vi "red_buoy_threshing_particle.vi"(4 "lum":cluster{"Lower value":i32, "Upper value":i32}={"Lower value"=0, "Upper value"=255}, 5 "hue":cluster{"Lower value":i32, "Upper value":i32}={"Lower value"=7, "Upper value"=14}, 6 "sat":cluster{"Lower value":i32, "Upper value":i32}={"Lower value"=0, "Upper value"=255}, 8 "Image":T1, 9 "error in (no error)":errorcluster) -> (0 "error out":errorcluster, 1 "circular particles":dbl[][](array[numeric]), 3 "Image Out":T1(plugin-control))   [LabVIEW 2009]
uses:
  <vilib>/vision/Image Controls.llb/IMAQ Image.ctl
  <vilib>/vision/NI_Vision_Development_Module.lvlib
panel:
  in  "max circularity":dbl
  out "size(s)":i32[](array[numeric])
  out "Particle Measurements (Pixels)":dbl[][](array[numeric]) format="%.2f"
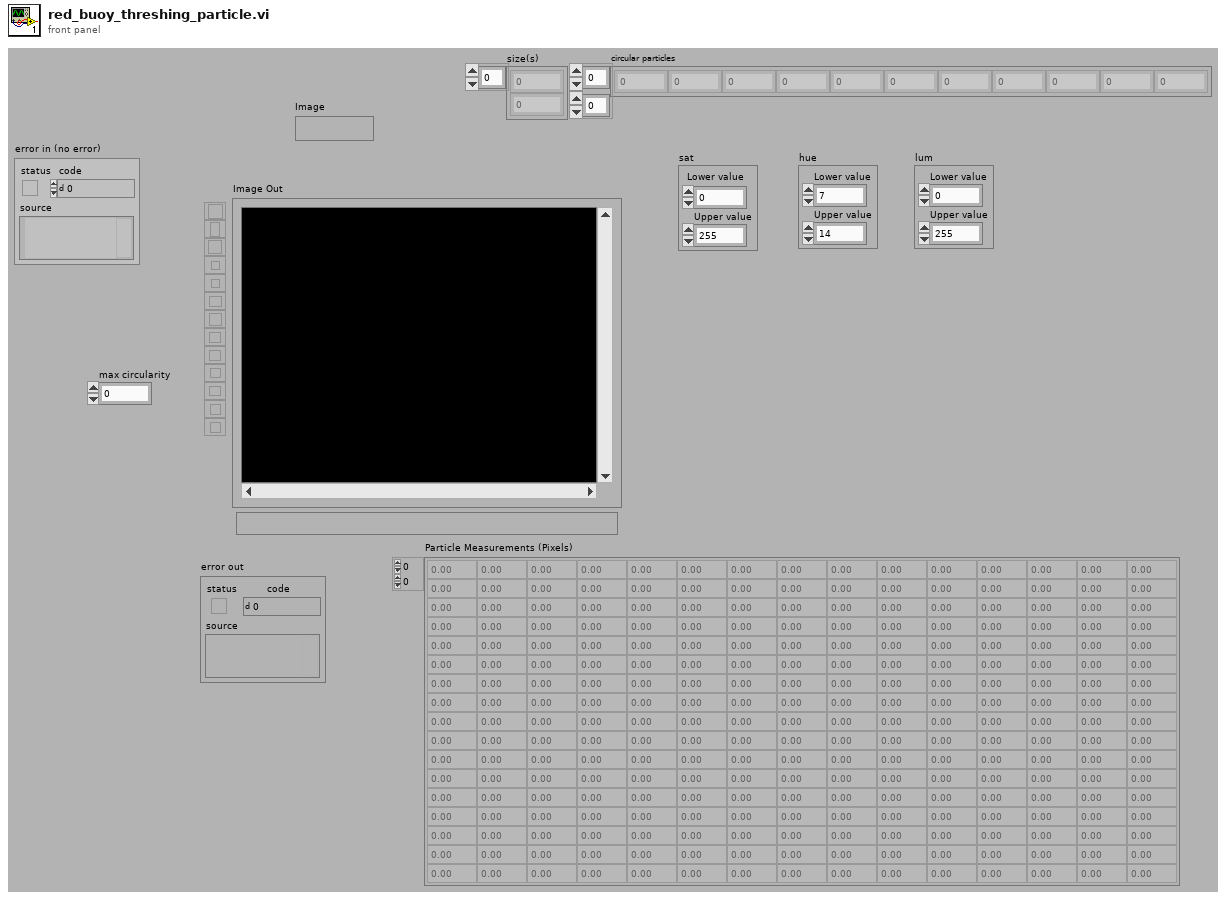
[diagram p1: front panel]
types:
  T1 = typedef "IMAQ Image.ctl" = refnum<image>
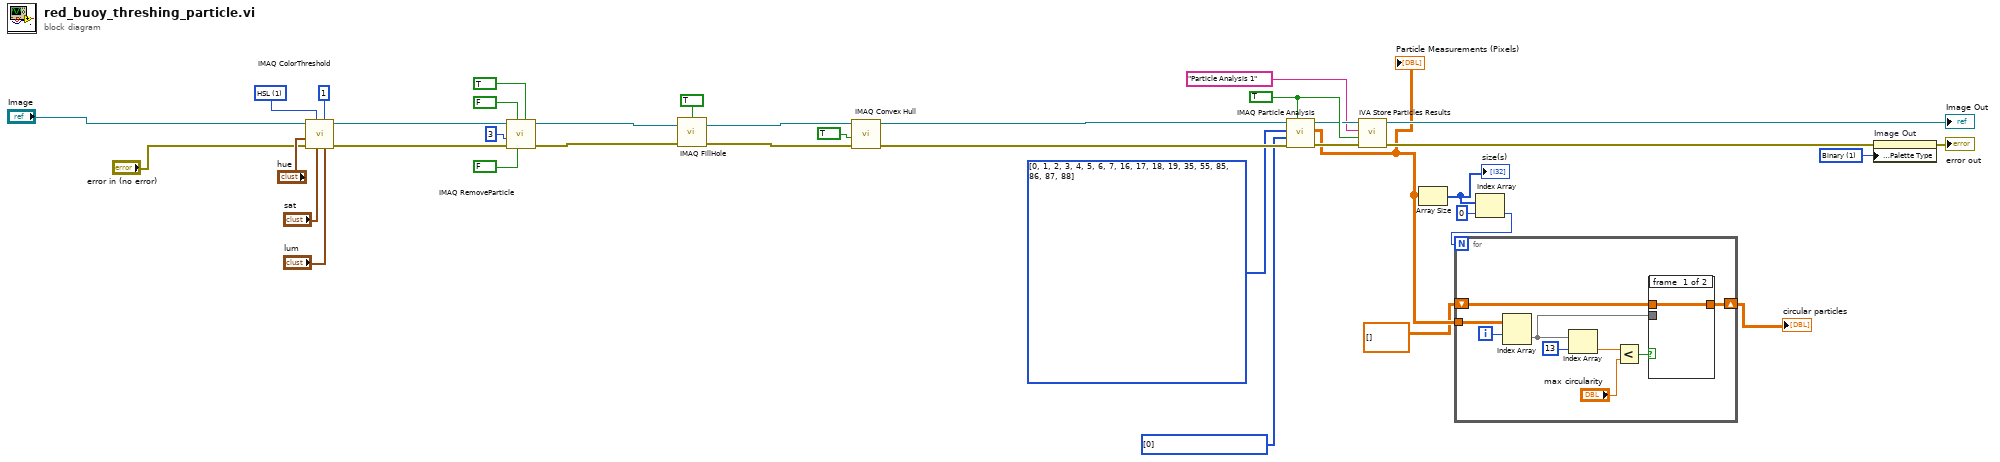
[diagram p0: block diagram]
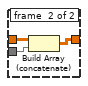
[diagram p2: hidden frame]
diagram:
  w11 = u32 1 items=["Grayscale", "Binary", "Gradient", "Rainbow", "Temperature", "User Defined"] ("Palette")
  w19 = i32[] [0] items=["Center of Mass X", "Center of Mass Y", "First Pixel X", "First Pixel Y", "Bounding Rect Left", "Bounding Rect Top", "Bounding Rect Right", "Bounding Rect Bottom", "Max Feret Diameter Start X", "Max Feret Diameter Start Y", "Max Feret Diameter End X", "Max Feret Diameter End Y", "Max Horiz. Segment Length Left", "Max Horiz. Segment Length Right", "Max Horiz. Segment Length Row", "-", "Bounding Rect Width", "Bounding Rect Height", "Bounding Rect Diagonal", "Perimeter", "Convex Hull Perimeter", "Holes' Perimeter", "Max Feret Diameter", "Equivalent Ellipse Major Axis", "Equivalent Ellipse Minor Axis", "Equivalent Ellipse Minor Axis (Feret)", "Equivalent Rect Long Side", "Equivalent Rect Short Side", "Equivalent Rect Diagonal", "Equivalent Rect Short Side (Feret)", "Average Horiz. Segment Length", "Average Vert. Segment Length", "Hydraulic Radius", "Waddel Disk Diameter", "-", "Area", "Holes' Area", "Particle & Holes' Area", "Convex Hull Area", "Image Area", "-", "Number of Holes", "Number of Horiz. Segments", "Number of Vert. Segments", "-", "Orientation", "Max Feret Diameter Orientation", "-", "% Area/Image Area", "% Area/(Particle & Holes' Area)", "Ratio of Equivalent Ellipse Axes", "Ratio of Equivalent Rect Sides", "-", "Elongation Factor", "Compactness Factor", "Heywood Circularity Factor", "Type Factor", "-", "Sum X", "Sum Y", "Sum XX", "Sum XY", "Sum YY", "Sum XXX", "Sum XXY", "Sum XYY", "Sum YYY", "-", "Moment of Inertia XX", "Moment of Inertia XY", "Moment of Inertia YY", "Moment of Inertia XXX", "Moment of Inertia XXY", "Moment of Inertia XYY", "Moment of Inertia YYY", "Norm. Moment of Inertia XX", "Norm. Moment of Inertia XY", "Norm. Moment of Inertia YY", "Norm. Moment of Inertia XXX", "Norm. Moment of Inertia XXY", "Norm. Moment of Inertia XYY", "Norm. Moment of Inertia YYY", "Hu Moment 1", "Hu Moment 2", "Hu Moment 3", "Hu Moment 4", "Hu Moment 5", "Hu Moment 6", "Hu Moment 7"] ("Real-World Measurements")
  w7 = i32[] [0, 1, 2, 3, 4, 5, 6, 7, 16, 17, 18, 19, 35, 55, 85, 86, 87, 88] items=["Center of Mass X", "Center of Mass Y", "First Pixel X", "First Pixel Y", "Bounding Rect Left", "Bounding Rect Top", "Bounding Rect Right", "Bounding Rect Bottom", "Max Feret Diameter Start X", "Max Feret Diameter Start Y", "Max Feret Diameter End X", "Max Feret Diameter End Y", "Max Horiz. Segment Length Left", "Max Horiz. Segment Length Right", "Max Horiz. Segment Length Row", "-", "Bounding Rect Width", "Bounding Rect Height", "Bounding Rect Diagonal", "Perimeter", "Convex Hull Perimeter", "Holes' Perimeter", "Max Feret Diameter", "Equivalent Ellipse Major Axis", "Equivalent Ellipse Minor Axis", "Equivalent Ellipse Minor Axis (Feret)", "Equivalent Rect Long Side", "Equivalent Rect Short Side", "Equivalent Rect Diagonal", "Equivalent Rect Short Side (Feret)", "Average Horiz. Segment Length", "Average Vert. Segment Length", "Hydraulic Radius", "Waddel Disk Diameter", "-", "Area", "Holes' Area", "Particle & Holes' Area", "Convex Hull Area", "Image Area", "-", "Number of Holes", "Number of Horiz. Segments", "Number of Vert. Segments", "-", "Orientation", "Max Feret Diameter Orientation", "-", "% Area/Image Area", "% Area/(Particle & Holes' Area)", "Ratio of Equivalent Ellipse Axes", "Ratio of Equivalent Rect Sides", "-", "Elongation Factor", "Compactness Factor", "Heywood Circularity Factor", "Type Factor", "-", "Sum X", "Sum Y", "Sum XX", "Sum XY", "Sum YY", "Sum XXX", "Sum XXY", "Sum XYY", "Sum YYY", "-", "Moment of Inertia XX", "Moment of Inertia XY", "Moment of Inertia YY", "Moment of Inertia XXX", "Moment of Inertia XXY", "Moment of Inertia XYY", "Moment of Inertia YYY", "Norm. Moment of Inertia XX", "Norm. Moment of Inertia XY", "Norm. Moment of Inertia YY", "Norm. Moment of Inertia XXX", "Norm. Moment of Inertia XXY", "Norm. Moment of Inertia XYY", "Norm. Moment of Inertia YYY", "Hu Moment 1", "Hu Moment 2", "Hu Moment 3", "Hu Moment 4", "Hu Moment 5", "Hu Moment 6", "Hu Moment 7"] ("Pixel Measurements")
  w17 = TRUE ("Connectivity 4/8 (8)")
  w36 = u16 1 items=["RGB", "HSL", "HSV", "HSI"] ("Color Mode")
  n1 = call "IMAQ ColorThreshold"("Blue or Luma or Val or Inten Range"="lum", "Replace Value"=1, "Green or Sat Range"="sat", "Color Mode"=w36, "error in (no error)"="error in (no error)", "Red or Hue Range"="hue", "Image Src"="Image") -> ("error out"=w32:errorcluster, "Image Dst Out"=w27:T1)  [unwired: 1 in, 2 out]
  n2 = call "IMAQ RemoveParticle"("Connectivity 4/8 (8)"=TRUE, "Low Pass/High Pass (Low)"=FALSE, "Square/Hexa (Square)"=FALSE, "error in (no error)"=w32, "Number of Erosion"=3, "Image Src"=w27) -> ("error out"=w26:errorcluster, "Image Dst Out"=w24:T1)  [unwired: 1 in, 3 out]
  n3 = call "IMAQ FillHole"("error in (no error)"=w26, "Image Src"=w24, "Connectivity 4/8 (8)"=TRUE) -> ("error out"=w23:errorcluster, "Image Dst Out"=w22:T1)  [unwired: 1 in, 2 out]
  n4 = call "IMAQ Convex Hull"("error in (no error)"=w23, "Connectivity 4/8 (8)"=TRUE, "Image Src"=w22) -> ("error out"=w20:errorcluster, "Image Dst Out"=w18:T1)  [unwired: 1 in, 6 out]
  n5 = call "IMAQ Particle Analysis"("Connectivity 4/8 (8)"=w17, "error in (no error)"=w20, "Real-World Measurements"=w19, "Pixel Measurements"=w7, "Image"=w18) -> ("error out"=w14:errorcluster, "Particle Measurements (Pixels)"=w6:dbl[][], "Image Out (duplicate)"=w16:T1)  [unwired: 4 out]
  "Particle Measurements (Pixels)" <- w6
  n6 = call <vilib>:"IVA Store Particles Results.vi"("error in (no error)"=w14, "Connectivity 4/8 (8)"=w17, "Step Name"="Particle Analysis 1", "Image in"=w16) -> ("error out"=w13:errorcluster, "Image dup"=→"Image Out":T1)  [unwired: 6 out]
  n7 = Array Size(array=w6) -> (size(s)=w5:i32[])
  "size(s)" <- w5
  n8 = Index Array(array=w5, index=0) -> (element=w3:i32)
  n9 = for {
    N: w3 -> [_]
    tunnel: w6 -> [w46]
    shift-right: [w38] -> w1
    shift-left: dbl[][] [] ("Particle Measurements (Pixels)") -> [w44]
    i -> [w45]
    n10 = Index Array(array=w46, index (row)=w45) -> (element=w39:dbl[])  [unwired: 1 in]
    n11 = Index Array(array=w39, index=13) -> (element=w42:dbl)
    n12 = Less?(x=w42, y="max circularity") -> (x < y?=w40:bool)
    n13 = case shown="True" w40 {
      tunnel: w44 -> [w47 w50]
      tunnel: w39 -> [_ w49]
      tunnel: [w47 w48] -> w38
      frame #0 {
      }
      frame #1 {
        n14 = Build Array (concatenate)(w50, w49) -> (w48:dbl[][])
      }
    }
  }
  "circular particles" <- w1
  n15 = property on="Image Out" class="ImageControl"(error in=w13, "Palette:Palette Type"=w11) -> (error out=→"error out":errorcluster)  [unwired: 1 in, 1 out]
